vi "OscilloscopeVI.vi"(8 "error in":errorcluster, 10 "ControlQueue":refnum<queue>, 11 "Oscilloscope.lvclass":refnum<class "Oscilloscope.lvclass">) -> (0 "error out":errorcluster)   [LabVIEW 2015, in "Oscilloscope.lvclass"]
doc: "This example shows how to use autosetup and acquire a waveform on a single channel for acquiring waveforms in a loop until stopped by user."
uses:
  Oscilloscope.lvclass
  dependecies/ControlsVIs/Clusters-def/Message types.ctl
  GeneralFunctionality/GeneralFunctionality.lvclass/GeneralFunctionality.ctl
  Message/Message.lvclass/Message.ctl
  dependecies/ControlsVIs/Clusters-def/Standard Command.ctl
  dependecies/ControlsVIs/Clusters-def/DAQmx-ELYSE_pulse_counter.ctl
  dependecies/ControlsVIs/Clusters-def/OSc-Demand-Read.ctl
  Message/Message.lvclass
  GeneralFunctionality/GeneralFunctionality.lvclass
  DAQmxTasks/DAQmxTaskContainer_General/DAQmxTaksContainer_General.lvclass
panel:
  out "Numeric":i32
  in  "Send to Det":bool
  in  "Channels":u16[](array[ring])=[0, 1] items=["Channel 1", "Channel 2", "Channel 3", "Channel 4"]
  out "ELYSE pulses":dbl
  in  "Timeout (10000 ms)":u32=10000
  in  "Read Osc":bool
  out "Received command":string
  out "Waveform Data":waveform(dbl)[](graph)
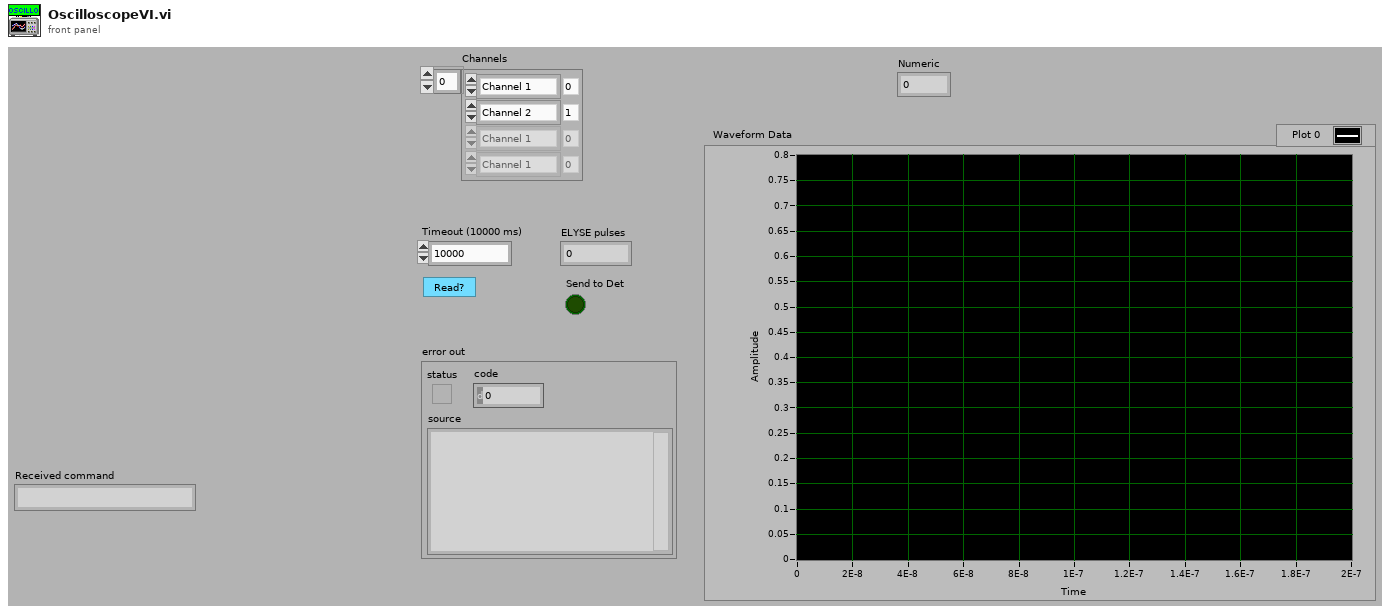
[diagram p1: front panel]
types:
  T1 = typedef "Message types.ctl" = string
  T2 = typedef "Standard Command.ctl" = cluster{"command":string, "data":variant}
  T3 = typedef "DAQmxTaksContainer_General.lvclass/DAQmx-ELYSE_pulse_counter.ctl" = cluster{"# counts":dbl}
  T4 = typedef "Oscilloscope.lvclass/OSc-Demand-Read.ctl" = cluster{"ON/OFF":bool, "Channels":u16[]}
  T5 = typedef "eventsource.ctl" = u32
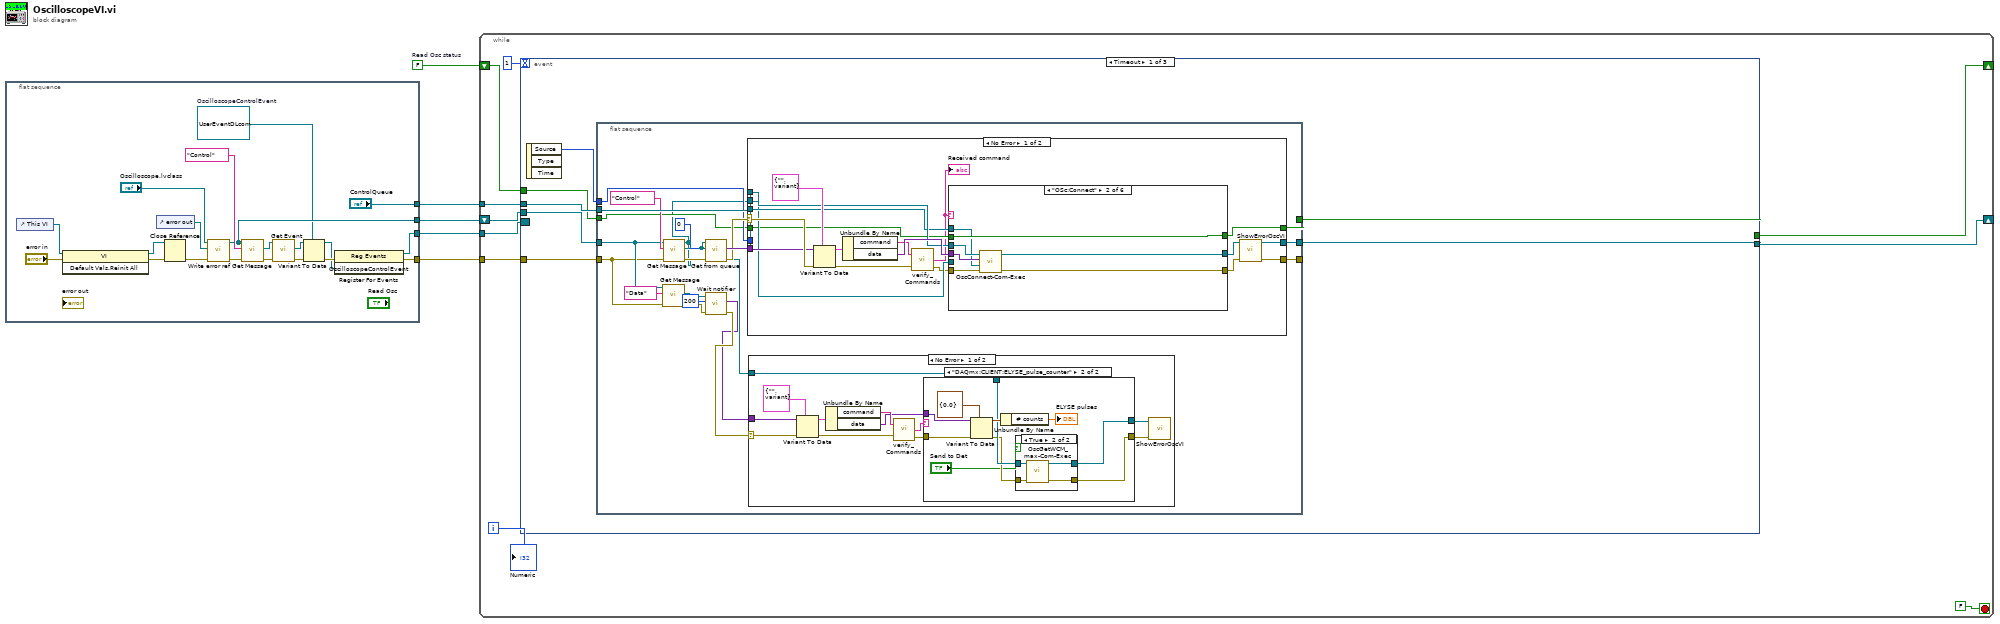
[diagram p0: block diagram]
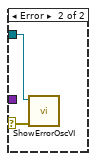
[diagram p4: hidden frame]
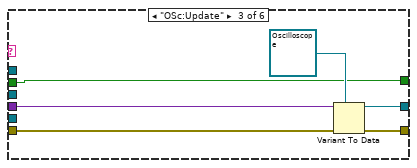
[diagram p6: hidden frame]
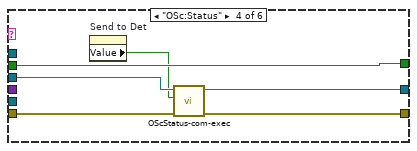
[diagram p7: hidden frame]
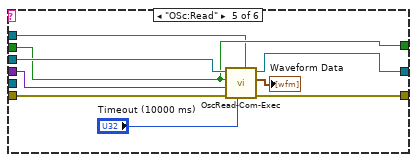
[diagram p8: hidden frame]
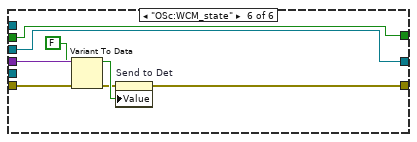
[diagram p9: hidden frame]
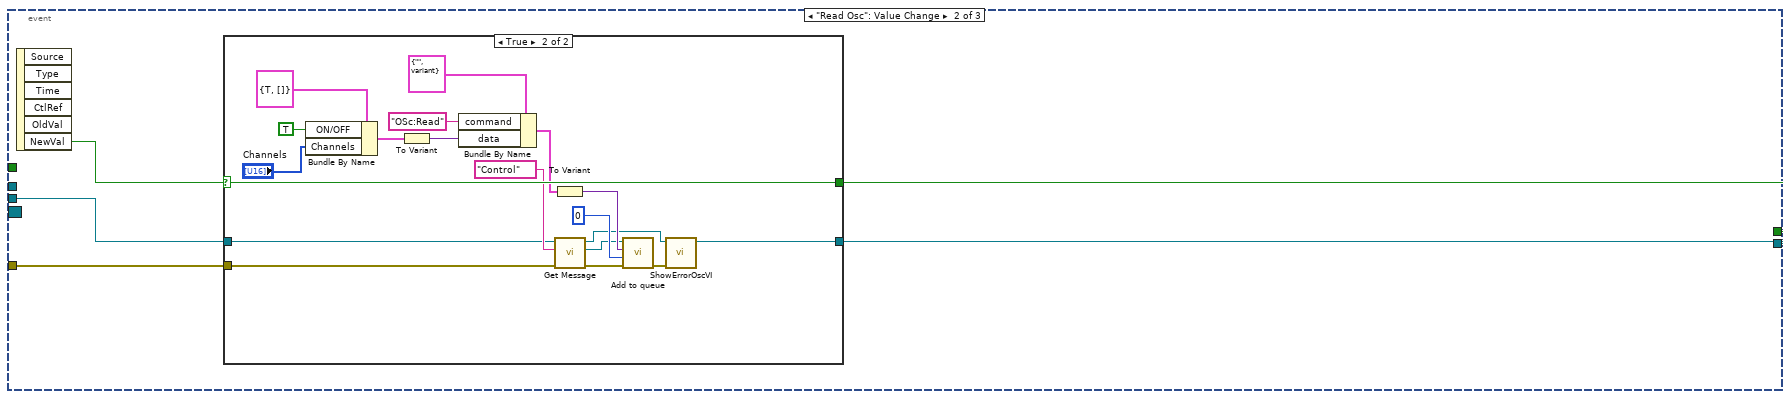
[diagram p11: hidden frame]
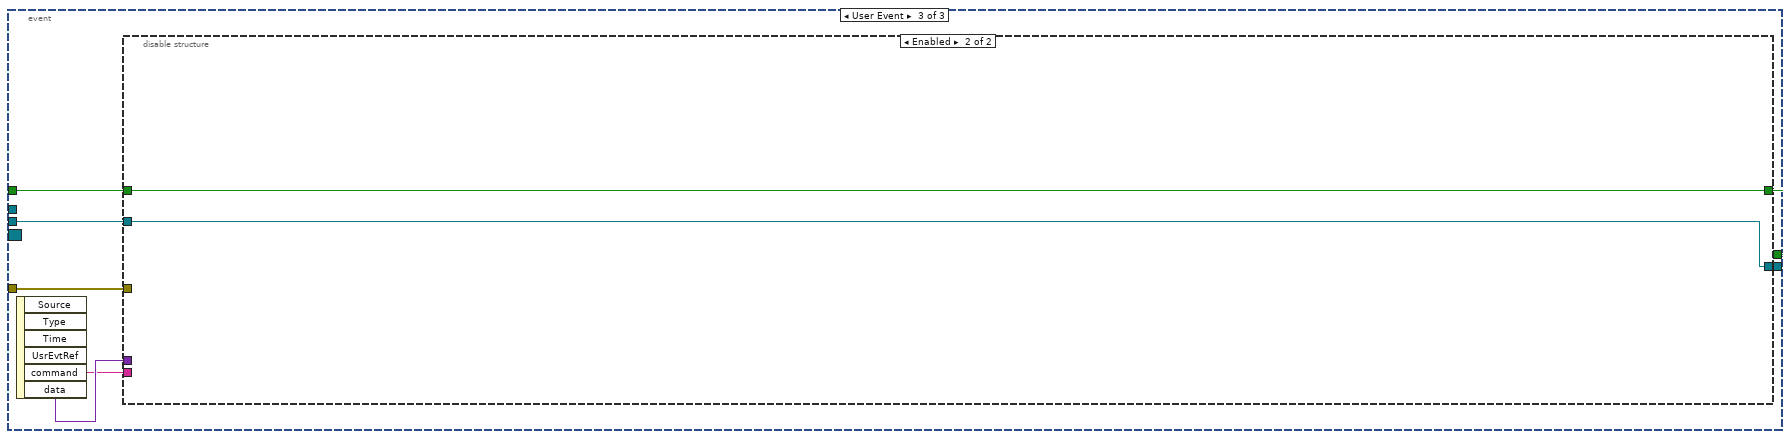
[diagram p13: hidden frame]
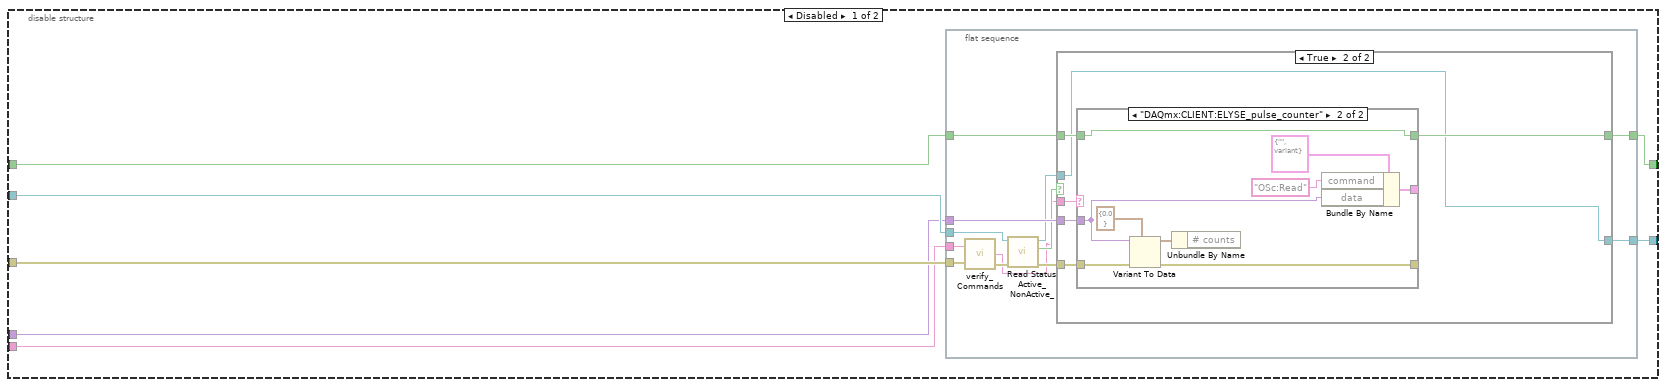
[diagram p14: hidden frame]
diagram:
  w2 = FALSE  # Read Osc status
  n1 = flat-sequence {
    tunnel: ["ControlQueue"] -> w5
    tunnel: [w19] -> w4
    tunnel: [w11] -> w3
    tunnel: [w12] -> w1
    frame #0 {
      w10 = refnum<user-event> refnum  # OscilloscopeControlEvent
      n2 = control-ref of="This VI"() -> (w23:refnum<vi>)
      n3 = invoke class="VI" method="Default Vals.Reinit All"(reference=w23, error in="error in") -> (reference out=w24:refnum<vi>, error out=w25:errorcluster)  [unwired: 1 in, 1 out]
      n4 = control-ref of="error out"() -> (w17:refnum<vi>)
      n5 = Close Reference(reference=w24, error in (no error)=w25) -> (error out=w16:errorcluster)
      n6 = call "Write error ref.vi"("error in (no error)"=w16, "error"=w17, "GeneralFunctionality in"="Oscilloscope.lvclass") -> ("error out"=w15:errorcluster, "GeneralFunctionality out"=w19:refnum<class "Oscilloscope.lvclass">)  [unwired: 7 in]
      n7 = call "Get Message.vi"("error in (no error)"=w15, "Message type"=T1 "Control", "GeneralFunctionality en entrée"=w19) -> ("error out"=w13:errorcluster, "Message.lvclass"=w14:refnum<class "Message.lvclass">)  [unwired: 6 in, 1 out]
      n8 = call "Get Event.vi"("error in (no error)"=w13, "Message en entrée"=w14) -> ("error out"=w9:errorcluster, "UserEventCommand"=w7:refnum<user-event>)  [unwired: 7 in, 1 out]
      n9 = Variant To Data(error in=w9, type=w10, Variant=w7) -> (data=w6:refnum<user-event>, error out=w8:errorcluster)
      n10 = register-events(error in=w8, w6) -> (reference out=w12:refnum<event-registration>, error out=w11:errorcluster)  [unwired: 1 in]
    }
  }
  n11 = while {
    tunnel: w5 -> [w34]
    tunnel: w3 -> [w31]
    shift-right: [w30] -> _
    shift-left: w4 -> [w32]
    shift-right: [w29] -> _
    shift-left: w2 -> [w28]
    tunnel: w1 -> [w27]
    i -> [w26]
    stop <- FALSE stop-if-true
    n12 = event shown="[0] Timeout" {
      selector: w27 -> [_ _ _]
      dyn-events: _ -> [_ _ _]
      timeout: 1 -> [_ _ _]
      tunnel: w34 -> [w42 _ _]
      tunnel: w32 -> [w40 w160 w188]
      tunnel: w31 -> [w39 w159 w187]
      tunnel: [w38 w158 w186] -> w30
      tunnel: [w36 w156 w184] -> w29
      tunnel: w28 -> [w37 _ w183]
      event Timeout {
        n13 = event-data() -> ("Source"=w41:T5)  [unwired: 1 in, 2 out]
        n14 = flat-sequence {
          tunnel: [w60] -> w38
          tunnel: [w59] -> _
          tunnel: w42 -> [w58]
          tunnel: [w57] -> w36
          tunnel: w41 -> [w56]
          tunnel: w40 -> [w51]
          tunnel: w39 -> [w50]
          tunnel: w37 -> [w52]
          frame #0 {
            n15 = call "Get Message.vi"("error in (no error)"=w50, "Message type"=T1 "Data", "GeneralFunctionality en entrée"=w51) -> ("error out"=w46:errorcluster, "Message.lvclass"=w47:refnum<class "Message.lvclass">)  [unwired: 6 in, 1 out]
            n16 = call "Get Message.vi"("error in (no error)"=w50, "Message type"=T1 "Control", "GeneralFunctionality en entrée"=w51) -> ("error out"=w55:errorcluster, "Message.lvclass"=w54:refnum<class "Message.lvclass">, "GeneralFunctionality en sortie"=w48:refnum<class "Oscilloscope.lvclass">)  [unwired: 6 in]
            n17 = call "Get from queue.vi"("error in (no error)"=w55, "timeout in ms (-1)"=0, "Message in"=w54) -> ("error out"=w61:errorcluster, "Data"=w62:variant)  [unwired: 6 in, 1 out]
            n18 = call "Wait notifier.vi"("error in (no error)"=w46, "timeout in ms (-1)"=200, "Message en entrée"=w47) -> ("error out"=w45:errorcluster, "notification"=w44:variant)  [unwired: 6 in, 1 out]
            n19 = case shown="No Error" w61 {
              selector: w61 -> [w113 w153]
              tunnel: w62 -> [w107 _]
              tunnel: [w103 w153] -> w59
              tunnel: w48 -> [w109 w154]
              tunnel: [w102 w154] -> w60
              tunnel: w58 -> [w108 _]
              tunnel: [w106 w155] -> w57
              tunnel: w54 -> [w105 _]
              tunnel: w56 -> [_ _]
              tunnel: w52 -> [w100 w155]
              frame No Error {
                n20 = Variant To Data(error in=w113, type=T2 {"command"="", "data"=variant} ("input cluster"), Variant=w107) -> (data=w111:T2, error out=w98:errorcluster)
                n21 = Unbundle By Name(w111) -> ("command"=w99:string, "data"=w110:variant)
                n22 = call "verify_Commands.vi"("Command"=w99, "error in"=w98) -> ("Command out"=w96:string, "error out"=w97:errorcluster)  [unwired: 1 out]
                "Received command" <- w96
                n23 = case shown="\"OSc:Connect\"" w96 {
                  tunnel: [w116 w122 w125 w132 w143 w147] -> w101
                  tunnel: [w115 w121 w127 w133 w142 w145] -> w104
                  tunnel: [w114 w119 w124 w135 w139 w148] -> w106
                  tunnel: w110 -> [_ w118 w129 _ w136 w152]
                  tunnel: w97 -> [w115 w120 w128 w134 w141 w151]
                  tunnel: w109 -> [w116 w123 _ w131 w144 w147]
                  tunnel: w108 -> [_ w117 _ _ w137 _]
                  tunnel: w105 -> [_ _ _ _ _ _]
                  tunnel: w100 -> [w114 w119 w124 w135 w139 w148]
                  frame "Error", Default {
                  }
                  frame "OSc:Connect" {
                    n24 = call "OscConnect-Com-Exec.vi"("error in (no error)"=w120, "ControlQueue"=w117, "data"=w118, "Oscilloscope in"=w123) -> ("error out"=w121:errorcluster, "Oscilloscope out"=w122:refnum<class "Oscilloscope.lvclass">)  [unwired: 6 in]
                  }
                  frame "OSc:Update" {
                    n25 = Variant To Data(error in=w128, type=refnum<class "Oscilloscope.lvclass"> refnum ("Oscilloscope.lvclass"), Variant=w129) -> (data=w125:refnum<class "Oscilloscope.lvclass">, error out=w127:errorcluster)
                  }
                  frame "OSc:Status" {
                    n26 = property on="Send to Det" class="Bool (strict)"() -> ("Value"=w130:bool)  [unwired: 2 in, 2 out]
                    n27 = call "OScStatus-com-exec.vi"("error in (no error)"=w134, "WCM_state"=w130, "Oscilloscope in"=w131) -> ("error out"=w133:errorcluster, "Oscilloscope out"=w132:refnum<class "Oscilloscope.lvclass">)  [unwired: 7 in]
                  }
                  frame "OSc:Read" {
                    n28 = call "OscRead-Com-Exec.vi"("ControlQueue"=w137, "Timeout (10000 ms)"="Timeout (10000 ms)", "error in (no error)"=w141, "data"=w136, "Multiple"=w139, "Oscilloscope in"=w144) -> ("error out"=w142:errorcluster, "Waveform Data OUT"=→"Waveform Data":waveform(dbl)[], "Oscilloscope out"=w143:refnum<class "Oscilloscope.lvclass">)  [unwired: 3 in]
                  }
                  frame "OSc:WCM_state" {
                    n29 = Variant To Data(error in=w151, type=FALSE, Variant=w152) -> (data=w149:bool, error out=w146:errorcluster)
                    n30 = property on="Send to Det" class="Bool (strict)"(error in=w146, "Value"=w149) -> (error out=w145:errorcluster)  [unwired: 1 in, 1 out]
                  }
                }
                n31 = call "ShowErrorOscVI.vi"("error in (no error)"=w104, "Oscilloscope in"=w101) -> ("error out"=w103:errorcluster, "Oscilloscope out"=w102:refnum<class "Oscilloscope.lvclass">)  [unwired: 8 in]
              }
              frame Error {
              }
            }
            n32 = case shown="No Error" w45 {
              selector: w45 -> [w73 w95]
              tunnel: w48 -> [w66 w94]
              tunnel: w44 -> [w64 _]
              frame No Error {
                n33 = Variant To Data(error in=w73, type=T2 {"command"="", "data"=variant} ("input cluster"), Variant=w64) -> (data=w75:T2, error out=w72:errorcluster)
                n34 = Unbundle By Name(w75) -> ("command"=w71:string, "data"=w67:variant)
                n35 = call "verify_Commands.vi"("Command"=w71, "error in"=w72) -> ("Command out"=w70:string, "error out"=w69:errorcluster)  [unwired: 1 out]
                n36 = case shown="\"DAQmx:CLIENT:ELYSE_pulse_counter\"" w70 {
                  tunnel: w69 -> [w77 w87]
                  tunnel: [w77 w79] -> w68
                  tunnel: w67 -> [_ w86]
                  tunnel: w66 -> [w76 w83]
                  tunnel: [w76 w82] -> w65
                  frame "Error", Default {
                  }
                  frame "DAQmx:CLIENT:ELYSE_pulse_counter" {
                    n37 = Variant To Data(error in=w87, type=T3 {"# counts"=0.0} ("OSc:Read"), Variant=w86) -> (data=w84:T3, error out=w81:errorcluster)
                    n38 = Unbundle By Name(w84) -> ("# counts"=→"ELYSE pulses":dbl)
                    n39 = case shown="True" "Send to Det" {
                      tunnel: w83 -> [w89 w93]
                      tunnel: [w89 w92] -> w82
                      tunnel: w81 -> [w88 w91]
                      tunnel: [w88 w90] -> w79
                      frame False {
                      }
                      frame True {
                        n40 = call "OscGetWCM_max-Com-Exec.vi"("error in (no error)"=w91, "Oscilloscope in"=w93) -> ("error out"=w90:errorcluster, "Oscilloscope out"=w92:refnum<class "Oscilloscope.lvclass">)  [unwired: 8 in]
                      }
                    }
                  }
                }
                n41 = call "ShowErrorOscVI.vi"("error in (no error)"=w68, "Oscilloscope in"=w65) -> ()  [unwired: 8 in, 2 out]
              }
              frame Error {
                n42 = call "ShowErrorOscVI.vi"("error in (no error)"=w95, "Oscilloscope in"=w94) -> ()  [unwired: 8 in, 2 out]
              }
            }
          }
        }
      }
      event "Read Osc": Value Change {
        n43 = event-data() -> ("NewVal"=w157:bool)  [unwired: 1 in, 5 out]
        n44 = case shown="True" w157 {
          selector: w157 -> [w162 w181]
          tunnel: [w162 w181] -> w156
          tunnel: w160 -> [w161 w171]
          tunnel: w159 -> [_ w170]
          tunnel: [w161 w167] -> w158
          frame False {
          }
          frame True {
            n45 = Bundle By Name(cluster=T4 {"ON/OFF"=TRUE, "Channels"=[]}, "ON/OFF"=TRUE, "Channels"="Channels") -> (w164:T4)
            n46 = To Variant(anything=w164) -> (Variant=w178:variant)
            n47 = Bundle By Name(cluster=T2 {"command"="", "data"=variant} ("command"), "command"="OSc:Read", "data"=w178) -> (w177:T2)
            n48 = To Variant(anything=w177) -> (Variant=w176:variant)
            n49 = call "Get Message.vi"("error in (no error)"=w170, "Message type"=T1 "Control", "GeneralFunctionality en entrée"=w171) -> ("error out"=w172:errorcluster, "Message.lvclass"=w173:refnum<class "Message.lvclass">, "GeneralFunctionality en sortie"=w168:refnum<class "Oscilloscope.lvclass">)  [unwired: 6 in]
            n50 = call "Add to queue.vi"("error in (no error)"=w172, "timeout in ms (-1)"=0, "Data"=w176, "Message in"=w173) -> ("error out"=w169:errorcluster)  [unwired: 6 in, 1 out]
            n51 = call "ShowErrorOscVI.vi"("error in (no error)"=w169, "Oscilloscope in"=w168) -> ("Oscilloscope out"=w167:refnum<class "Oscilloscope.lvclass">)  [unwired: 8 in, 1 out]
          }
        }
      }
      event User Event {
        n52 = event-data() -> ("command"=w182:string, "data"=w185:variant)  [unwired: 1 in, 4 out]
        n53 = disable-structure shown="Enabled" {
          disable-tunnel: w188 -> [w195 w227]
          disable-tunnel: w187 -> [w194 _]
          disable-tunnel: [w193 w227] -> w186
          disable-tunnel: w185 -> [w192 _]
          disable-tunnel: [w191 w228] -> w184
          disable-tunnel: w183 -> [w190 w228]
          disable-tunnel: w182 -> [w189 _]
          frame Disabled {
            n54 = flat-sequence {
              tunnel: w195 -> [w202]
              tunnel: w194 -> [w198]
              tunnel: [w204] -> w193
              tunnel: w192 -> [w207]
              tunnel: [w206] -> w191
              tunnel: w190 -> [w205]
              tunnel: w189 -> [w199]
              frame #0 {
                n55 = call "verify_Commands.vi"("Command"=w199, "error in"=w198) -> ("Command out"=w196:string, "error out"=w197:errorcluster)  [unwired: 1 out]
                n56 = call "Read Status Active_NonActive_.vi"("error in (no error)"=w197, "Oscilloscope in"=w202) -> ("error out"=w201:errorcluster, "Status Active/NonActive"=w203:bool, "Oscilloscope out"=w200:refnum<class "Oscilloscope.lvclass">)  [unwired: 7 in]
                n57 = case shown="True" w203 {
                  tunnel: w207 -> [_ w215]
                  tunnel: [w208 w214] -> w206
                  tunnel: w205 -> [w208 w213]
                  tunnel: w201 -> [_ w212]
                  tunnel: w196 -> [_ w211]
                  tunnel: [w209 w210] -> w204
                  tunnel: w200 -> [w209 w210]
                  frame False {
                  }
                  frame True {
                    n58 = case shown="\"DAQmx:CLIENT:ELYSE_pulse_counter\"" w211 {
                      tunnel: [_ w225] -> _
                      tunnel: w215 -> [_ w221]
                      tunnel: [w217 w218] -> w214
                      tunnel: w213 -> [w217 w218]
                      tunnel: w212 -> [w216 w223]
                      tunnel: [w216 w222] -> _
                      frame "Faux", Default {
                      }
                      frame "DAQmx:CLIENT:ELYSE_pulse_counter" {
                        n59 = Variant To Data(error in=w223, type=T3 {"# counts"=0.0} ("OSc:Read"), Variant=w221) -> (data=w220:T3, error out=w222:errorcluster)
                        n60 = Unbundle By Name(w220) -> ()  [unwired: 1 out]
                        n61 = Bundle By Name(cluster=T2 {"command"="", "data"=variant} ("command"), "command"="OSc:Read", "data"=w221) -> (w225:T2)
                      }
                    }
                  }
                }
              }
            }
          }
          frame Enabled {
          }
        }
      }
    }
    "Numeric" <- w26
  }
